vi "GT Get Capture Status.vi"(0 "cardNum":i16, 1 "count":i16, 5 "encoder":i16, 7 "pStatus":i16, 9 "pValue":i32, 11 "error in (no error)":errorcluster caption="错误输入（无错误）", 12 "pClock":u32) -> (4 "function return":i16, 8 "pStatus out":i16, 10 "pValue out":i32, 14 "pClock out":u32, 15 "error out":errorcluster caption="错误输出")   [LabVIEW 2020, in "gts.lvlib"]
doc: "GT_API GT_GetCaptureStatus(short cardNum,short encoder,short *pStatus,long *pValue,short count=1,unsigned long *pClock=NULL);"
uses:
  gts.lvlib
  dll/32bit/multi_card/gts.dll
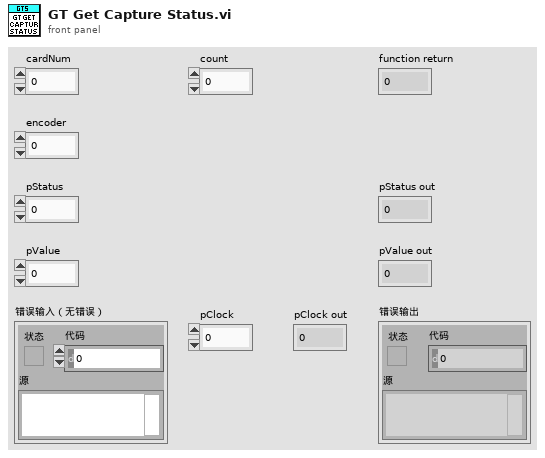
[diagram p1: front panel]
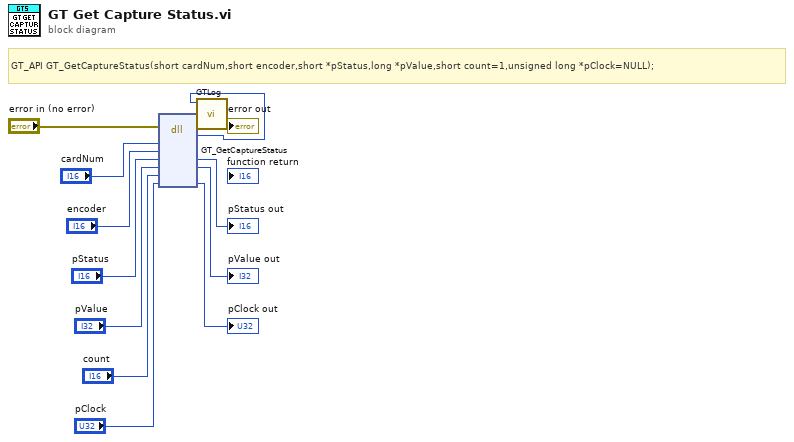
[diagram p0: block diagram]
diagram:
  # "GT_API GT_GetCaptureStatus(short cardNum,short encoder,short *pStatus,long *pValue,short count=1,unsigned long *pClock=NULL);"
  n1 = dll-call lib="C:/1228/dll/32bit/multi_card/gts.dll" fn="GT_GetCaptureStatus"(error in="error in (no error)", "cardNum"="cardNum", "encoder"="encoder", "pStatus"="pStatus", "pValue"="pValue", "count"="count", "pClock"="pClock") -> (error out=w3:errorcluster, "返回类型"=w1:i16, "pStatus"=→"pStatus out":i16, "pValue"=→"pValue out":i32, "pClock"=→"pClock out":u32)  [unwired: 5 in, 1 out]
  n2 = call "GTLog.vi"("error in (no error)"=w3, "Numeric"=w1) -> ("error out"=→"error out":errorcluster)  [unwired: 9 in]
